vi "Display the Learning Curve.vi"() -> ()   [LabVIEW 2023]
doc: "This example demonstrates how to plot the learning curve of an adaptive filter. The learning curve shows the mean square error (MSE) of the error signal over a specified number of iterations. You can use the learning curve to evaluate performance aspects of an adaptive filter, including the convergence speed and steady state error.\n\nThis example computes the error signal with a number of trials and then calculates the MSE of the error signal. \n\nComplete the following steps to use this example:\n\n1. Run this VI. \n\n2. Select an adaptive filter algorithm and set values for its parameters.\n\n3. Click the <b>Compute</b> button to compute the learning curve."
uses:
  <vilib>/addons/Adaptive Filters/Create/AFT Create FIR LMS (Real).vi
  <vilib>/addons/Adaptive Filters/Create/AFT Create FIR Normalized LMS (Real).vi
  <vilib>/addons/Adaptive Filters/Create/AFT Create FIR RLS (Real).vi
  <vilib>/addons/Adaptive Filters/Create/AFT Create FIR QR-RLS (Real).vi
  <vilib>/addons/Adaptive Filters/Processing/AFT Filter Signal and Update Coefficients (Real, Array).vi
  <vilib>/addons/Adaptive Filters/NI_AdaptiveFilter.lvlib
panel:
  in  "Stop":bool
  out "Parameter Selection":T1(tab)
  in  "LMS Step Size":dbl=0.02 min=0.0 step=0.01
  in  "NLMS Step Size":dbl=0.5 min=0.0 max=2.0 step=0.1
  in  "Sign LMS Step Size":dbl=0.005 min=0.0 step=0.001
  in  "RLS \nForgetting Factor":dbl=0.95 min=0.0 max=1.0 step=0.01
  in  "QR-RLS \nForgetting Factor":dbl=0.95 min=0.0 max=1.0 step=0.01
  in  "Compute":bool
  in  "Samples":i32=1000 min=100
  in  "Algorithm":T2(ring)
  in  "Trials":i32=100 min=1
  out "Learning Curve":dbl[](graph)
  # "Select Help>>Show Context Help and move the cursor over the VI icon of this example for more information."
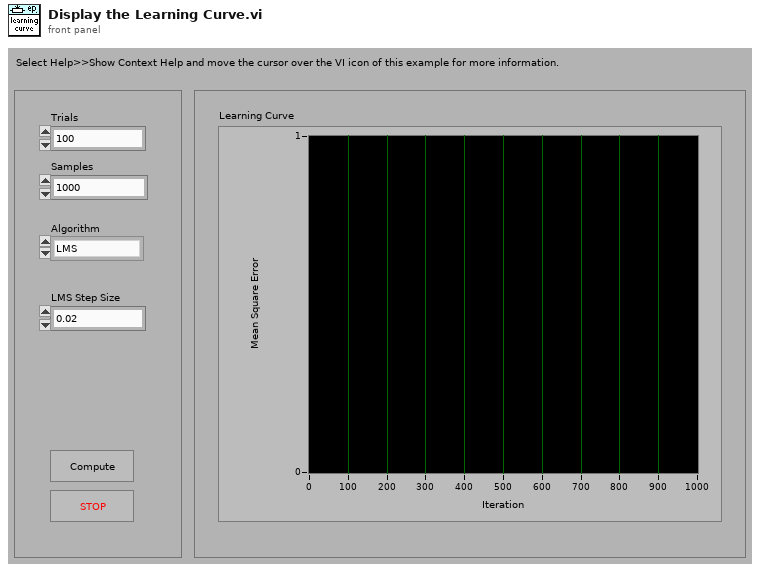
[diagram p1: front panel]
types:
  T1 = enum32{"LMS", "Normalized LMS", "Sign LMS", "RLS", "QR-RLS"}
  T2 = enum16{"LMS", "Normalized LMS", "Sign LMS", "RLS", "QR-RLS"}
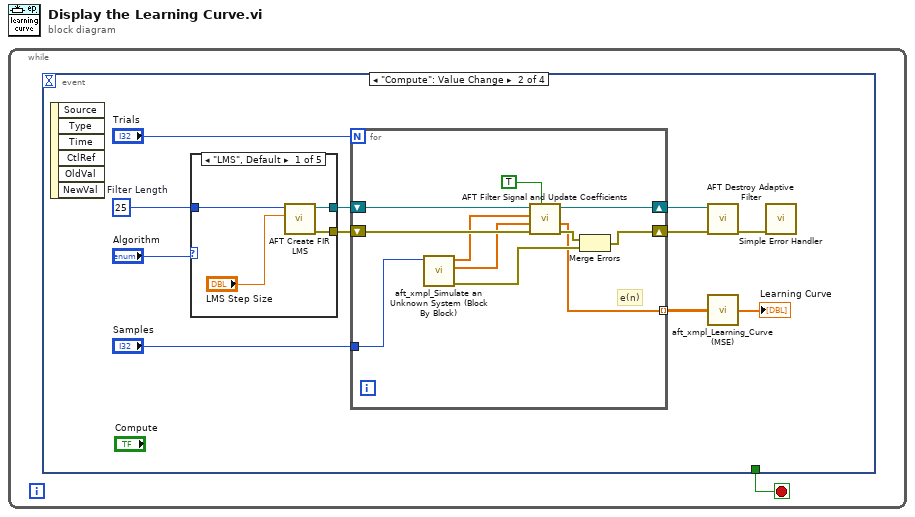
[diagram p0: block diagram]
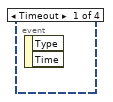
[diagram p2: hidden frame]
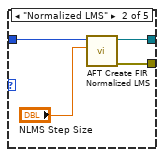
[diagram p3: hidden frame]
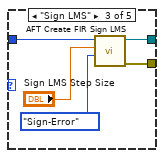
[diagram p4: hidden frame]
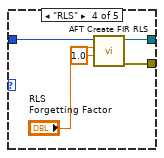
[diagram p5: hidden frame]
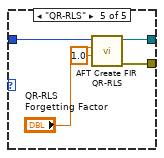
[diagram p6: hidden frame]
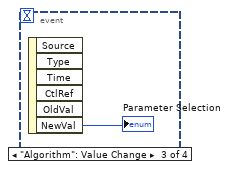
[diagram p7: hidden frame]
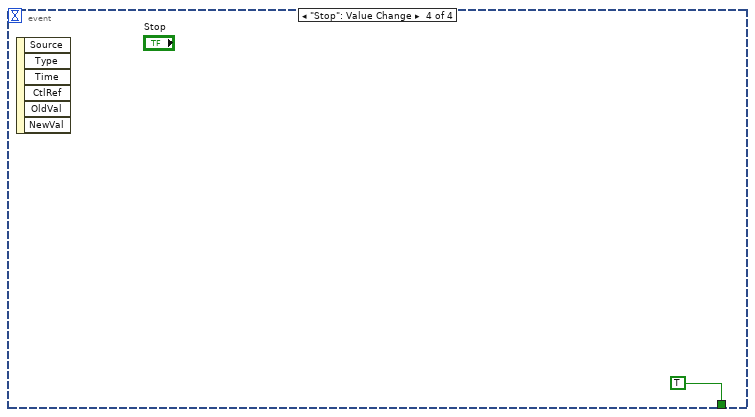
[diagram p8: hidden frame]
diagram:
  n1 = while {
    stop <- w1 stop-if-true
    n2 = event shown="[1] \"Compute\": Value Change" {
      selector: _ -> [_ _ _ _]
      dyn-events: _ -> [_ _ _ _]
      timeout: _ -> [_ _ _ _]
      tunnel: [_ _ _ TRUE] -> w1
      event Timeout {
        n3 = event-data() -> ()  [unwired: 3 out]
      }
      event "Compute": Value Change {
        w11 = 25  # Filter Length
        n4 = event-data() -> ()  [unwired: 7 out]
        n5 = case shown="\"LMS\", Default" "Algorithm" {
          tunnel: w11 -> [w16 w18 w23 w28 w33]
          tunnel: [w15 w20 w25 w30 w35] -> w10
          tunnel: [w14 w19 w24 w29 w34] -> w9
          frame "LMS", Default {
            n6 = call-poly <vilib>:"AFT Create FIR LMS.vi"("step size"="LMS Step Size", "filter length"=w16) -> ("error out"=w14:errorcluster, "adaptive filter out"=w15:refnum<k20>)  [unwired: 2 in, 6 out]
          }
          frame "Normalized LMS" {
            n7 = call-poly <vilib>:"AFT Create FIR Normalized LMS.vi"("step size"="NLMS Step Size", "filter length"=w18) -> ("error out"=w19:errorcluster, "adaptive filter out"=w20:refnum<k20>)  [unwired: 2 in, 6 out]
          }
          frame "Sign LMS" {
            n8 = call <vilib>:"AFT Create FIR Sign LMS.vi"("sign type"=enum16{"Sign-Error", "Sign-Data", "Sign-Sign"}."Sign-Error", "step size"="Sign LMS Step Size", "filter length"=w23) -> ("error out"=w24:errorcluster, "adaptive filter out"=w25:refnum<k20>)  [unwired: 1 in, 6 out]
          }
          frame "RLS" {
            n9 = call-poly <vilib>:"AFT Create FIR RLS.vi"("regularization factor"=1.0, "forgetting factor"="RLS \nForgetting Factor", "filter length"=w28) -> ("error out"=w29:errorcluster, "adaptive filter out"=w30:refnum<k20>)  [unwired: 1 in, 6 out]
          }
          frame "QR-RLS" {
            n10 = call-poly <vilib>:"AFT Create FIR QR-RLS.vi"("regularization factor"=1.0, "forgetting factor"="QR-RLS \nForgetting Factor", "filter length"=w33) -> ("error out"=w34:errorcluster, "adaptive filter out"=w35:refnum<k20>)  [unwired: 1 in, 6 out]
          }
        }
        n11 = for {
          N: "Trials" -> [_]
          tunnel: "Samples" -> [w42]
          shift-right: [w43] -> w8
          shift-left: w10 -> [w46]
          shift-right: [w37] -> w7
          shift-left: w9 -> [w45]
          tunnel: [w36] -> w6 mode=indexing
          # "e(n)"
          n12 = call "aft_xmpl_Simulate an Unknown System (Block By Block).vi"("samples"=w42) -> ("error out"=w38:errorcluster, "response signal"=w40:dbl[], "stimulus signal"=w41:dbl[])  [unwired: 3 in, 5 out]
          n13 = call-poly <vilib>:"AFT Filter Signal and Update Coefficients.vi"("reset? (F)"=TRUE, "error in (no error)"=w45, "d(n)"=w40, "x(n)"=w41, "adaptive filter in"=w46) -> ("error out"=w39:errorcluster, "e(n)"=w36:dbl[], "adaptive filter out"=w43:refnum<k20>)  [unwired: 1 in, 3 out]
          n14 = Merge Errors(w39, w38) -> (w37:errorcluster)
        }
        n15 = call <vilib>:"AFT Destroy Adaptive Filter.vi"("error in (no error)"=w7, "adaptive filter in"=w8) -> ("error out"=w2:errorcluster)  [unwired: 9 out]
        n16 = call "aft_xmpl_Learning_Curve (MSE).vi"("e(n)"=w6) -> ("MSE"=→"Learning Curve":dbl[])
        n17 = call <vilib>:"Simple Error Handler.vi"("error in (no error)"=w2) -> ()  [unwired: 1 in, 8 out]
      }
      event "Algorithm": Value Change {
        n18 = event-data() -> ("NewVal"=→"Parameter Selection":T2)  [unwired: 6 out]
      }
      event "Stop": Value Change {
        n19 = event-data() -> ()  [unwired: 7 out]
      }
    }
  }
